vi "LRU Add.vi"(10 "Value":u64, 11 "State":cluster{"Hallway":string[], "Rooms":string[][]}) -> ()   [LabVIEW 2019, in "23.lvlib"]
uses:
  23.lvlib
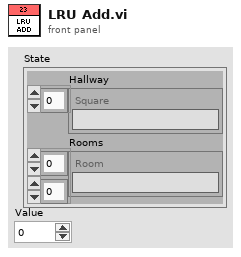
[diagram p1: front panel]
types:
  T1 = cluster{"Stop":bool, "Check":bool, "Key":cluster{"Hallway":string[], "Rooms":string[][]}, "Value":u64, "Check Notifier":refnum<notifier>}
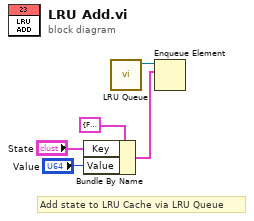
[diagram p0: block diagram]
diagram:
  # "Add state to LRU Cache via LRU Queue"
  n1 = Bundle By Name(cluster=T1 {"Stop"=FALSE, "Check"=FALSE, "Key"={"Hallway"=[], "Rooms"=[]}, "Value"=0, "Check Notifier"=refnum}, "Key"="State", "Value"="Value") -> (w4:T1)
  n2 = call "LRU Queue.vi"() -> ("LRU Queue"=w3:refnum<queue>)  [unwired: 11 in]
  n3 = Enqueue Element(queue=w3, element=w4) -> ()  [unwired: 2 in, 3 out]
